vi "ExSubSpecOpenIndex.vi"(3 "error in (no error)":errorcluster, 4 "Grating speed":dbl format="%.2f", 5 "Grating number":i16, 6 "Index":i16) -> (0 "error out":errorcluster, 1 "Camera Handle":u32, 2 "Spectrometer Handle":u32)   [LabVIEW 2010]
panel:
  in  "Camera Handle":u32
  # "ExSubSpecOpenIndex:\nThis Sub-VI opens a spectrometer based on\nan Index, sets the grating and sets the speed\nfor wavelength movement. It returns a\nspectrometer handle.  An index of 0 uses the\ndefault spectrometer which is the first one\nlisted in the first .ini file found."
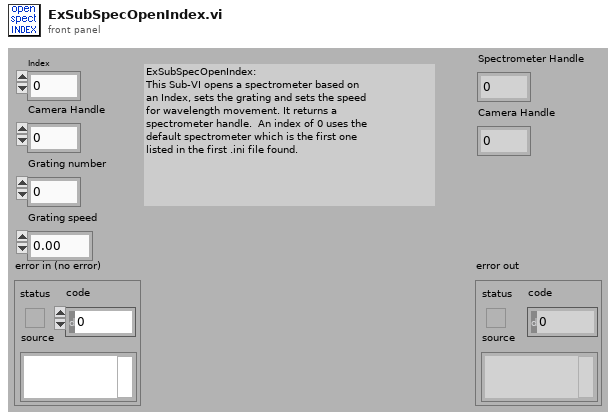
[diagram p1: front panel]
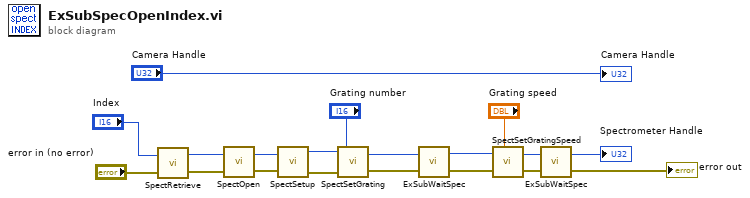
[diagram p0: block diagram]
diagram:
  n1 = call <userlib>:"SpectRetrieve.vi"("error in"="error in (no error)", "Index"="Index") -> ("error out"=w3:errorcluster, "Device ID"=w2:u32)
  n2 = call <userlib>:"SpectOpen.vi"("error in"=w3, "Spectrometer ID"=w2) -> ("error out"=w6:errorcluster, "Spectrometer Handle"=w8:u32)  [unwired: 1 in]
  n3 = call <userlib>:"SpectSetup.vi"("error in"=w6, "Spectrometer Handle"=w8) -> ("error out"=w5:errorcluster, "Spectrometer Handle"=w7:u32)
  n4 = call <userlib>:"SpectSetGrating.vi"("error in"=w5, "Grating Number"="Grating number", "Sepctrometer Handle"=w7) -> ("error out"=w16:errorcluster, "Spectrometer Handle"=w15:u32)
  n5 = call "ExSubWaitSpec.vi"("error in (no error)"=w16, "Spectrometer Handle"=w15) -> ("error out"=w14:errorcluster, "Spectrometer handle"=w13:u32)
  n6 = call <userlib>:"SpectSetGratingSpeed.vi"("error in"=w14, "Grating Speed"="Grating speed", "Spectrometer Handle"=w13) -> ("error out"=w11:errorcluster, "Spectrometer Handle"=w12:u32)
  n7 = call "ExSubWaitSpec.vi"("error in (no error)"=w11, "Spectrometer Handle"=w12) -> ("error out"=→"error out":errorcluster, "Spectrometer handle"=→"Spectrometer Handle":u32)
  "Camera Handle" <- "Camera Handle"
